vi "getVariaControls.vi"(6 "error in (no error)":errorcluster, 9 "COMport":string="COM6") -> (0 "error out":errorcluster, 1 "LPFilterSetpointAngstrom":u16, 2 "SWFilterSetpointAngstrom":u16, 3 "NDFilterSetpointPercentx10":u16)   [LabVIEW 2015]
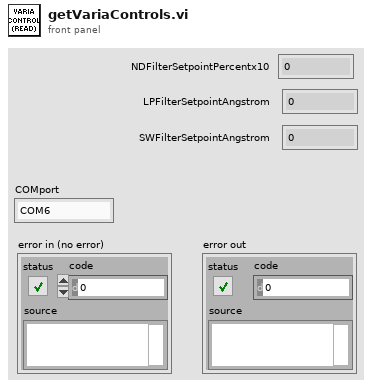
[diagram p1: front panel]
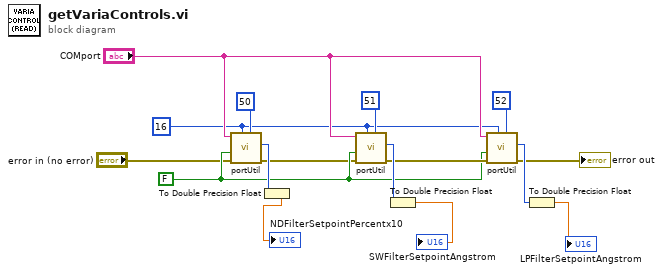
[diagram p0: block diagram]
diagram:
  w5 = FALSE ("WriteNotRead")
  w3 = u8 16 ("Destination")
  n1 = call "portUtil.vi"("Register"=u8 50, "Destination"=w3, "error in (no error)"="error in (no error)", "WriteNotRead"=w5, "COMport"="COMport") -> ("error out"=w1:errorcluster, "Long"=w7:i32)  [unwired: 4 in, 1 out]
  n2 = To Double Precision Float(number=w7) -> (double precision float=→"NDFilterSetpointPercentx10":dbl)
  n3 = call "portUtil.vi"("Register"=u8 51, "Destination"=w3, "error in (no error)"=w1, "WriteNotRead"=w5, "COMport"="COMport") -> ("error out"=w12:errorcluster, "Long"=w15:i32)  [unwired: 4 in, 1 out]
  n4 = To Double Precision Float(number=w15) -> (double precision float=→"SWFilterSetpointAngstrom":dbl)
  n5 = call "portUtil.vi"("Register"=u8 52, "Destination"=w3, "error in (no error)"=w12, "WriteNotRead"=w5, "COMport"="COMport") -> ("error out"=→"error out":errorcluster, "Long"=w13:i32)  [unwired: 4 in, 1 out]
  n6 = To Double Precision Float(number=w13) -> (double precision float=→"LPFilterSetpointAngstrom":dbl)
